vi "End NI_XNET_CAN_Bus_Monitor_API StreamBus.vi"(8 "error in":errorcluster, 10 "Cancel All Reads (F)":bool, 11 "Call ID in":T2) -> (0 "error out":errorcluster, 1 "errorDetails":T1)   [LabVIEW 2025, in "xnet_can_bus_monitor_api_client.lvlib"]
uses:
  xnet_can_bus_monitor_api_client.lvlib
  <vilib>/gRPC/LabVIEW gRPC Library/Shared/grpcId.ctl
  <vilib>/gRPC/LabVIEW gRPC Library/Shared/Any.ctl
  <vilib>/gRPC/LabVIEW gRPC Library/grpc-lvsupport-release.lvlib
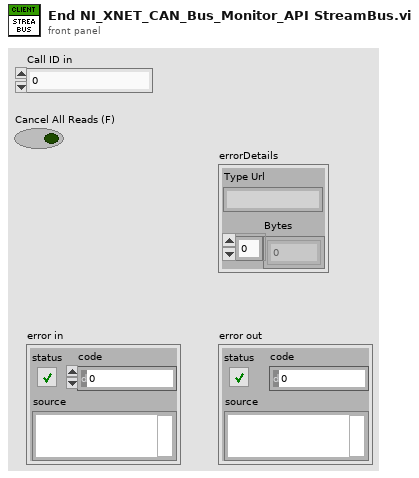
[diagram p1: front panel]
types:
  T1 = typedef "grpc-lvsupport-release.lvlib/Any.ctl" = cluster{"Type Url":string, "Bytes":u8[]}
  T2 = typedef "grpc-lvsupport-release.lvlib/grpcId.ctl" = u64
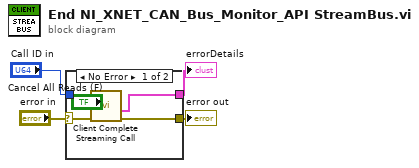
[diagram p0: block diagram]
diagram:
  n1 = case shown="No Error" "error in" {
    selector: "error in" -> [w9 w10]
    tunnel: [w8 w10] -> w3
    tunnel: "Call ID in" -> [w7 _]
    tunnel: [w6 _] -> w1
    frame No Error {
      n2 = call <vilib>:"Client Complete Streaming Call.vi"("error in"=w9, "Cancel All Reads (F)"="Cancel All Reads (F)", "Call ID in"=w7) -> ("error out"=w8:errorcluster, "errorDetails"=w6:T1)  [unwired: 7 in]
    }
    frame Error {
    }
  }
  "error out" <- w3
  "errorDetails" <- w1
